vi "Get Card Model.vi"(8 "error in (no error)":errorcluster, 9 "Slot Number":u32, 11 "VISA resource name":refnum<visa-resource-name>) -> (0 "error out":errorcluster, 1 "Card Model":string, 3 "VISA resource name out":refnum<visa-resource-name>)   [LabVIEW 2018, in "Keithley 3706.lvlib"]
uses:
  <instrlib>/Keithley 3706/Keithley 3706.lvlib
panel:
  out "x = y?":bool
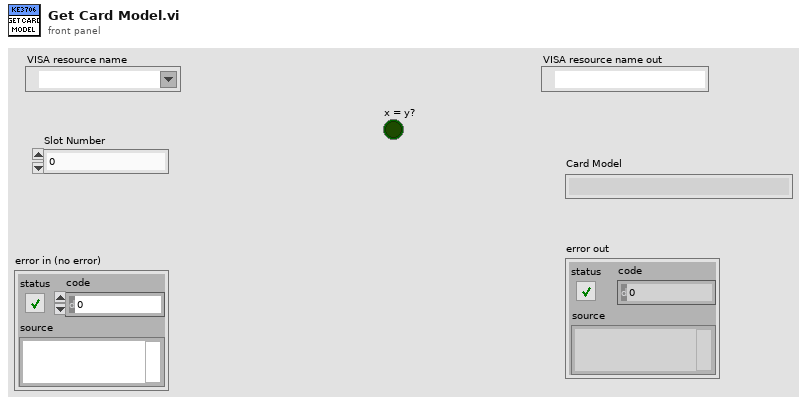
[diagram p1: front panel]
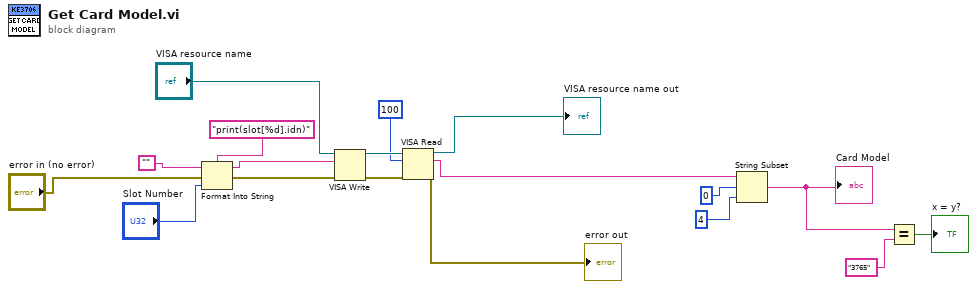
[diagram p0: block diagram]
diagram:
  n1 = Format Into String(format string="print(slot[%d].idn)", initial string="", error in="error in (no error)", "Slot Number") -> (resulting string=w12:string, error out=w14:errorcluster)
  n2 = VISA Write(VISA resource name="VISA resource name", write buffer=w12, error in (no error)=w14) -> (VISA resource name out=w11:refnum<visa-resource-name>, error out=w10:errorcluster)  [unwired: 1 out]
  n3 = VISA Read(VISA resource name=w11, byte count=100, error in (no error)=w10) -> (VISA resource name out=→"VISA resource name out":refnum<visa-resource-name>, read buffer=w5:string, error out=→"error out":errorcluster)  [unwired: 1 out]
  n4 = String Subset(string=w5, offset (0)=0, length (rest)=4) -> (substring=w3:string)
  "Card Model" <- w3
  n5 = Equal?(x=w3, y="3765") -> (x = y?=→"x = y?":bool)
